vi "SVPO Vector Average Spectrum (Complex) (1 Ch).vi"(0 "complex spectrum [EU rms]":T7={"complex spectrum response"={"f0"=0.0, "df"=1.0, "complex spectrum"=[]}, "spectrum info"={"channel name"="", "description"="", "x-axis units"=0, "spectral info"={"spectrum type"=enum."Power [Magnitude^2]", "linear/dB"=enum."linear", "window"=0, "window size"=0, "FFT size"=0}, "engineering units"=0, "custom label"="", "dB reference [EU]"=0.0, "peak units"=enum."rms", "weighting filter"=0, "spectral density?"=FALSE, "unit label"="", "spectrum skewed?"=FALSE, "complimentary spectrum units"=enum."none"}} {"spectrum info"."x-axis units" items=["Time (s)"=0, "Frequency-CB (Hz)"=1, "Frequency-CPB (Hz)"=1248, "Frequency-Arbitrary (Hz)"=2357, "Quefrency (s)"=2, "Revolutions (rev)"=3, "Order"=4, "Speed (RPM)"=11, "Speed (rad/s)"=21, "Index"=65535]; "spectrum info"."weighting filter" items=["Linear", "A-weighting", "B-weighting", "C-weighting", "ITU-R 468-4", "Dolby", "CCITT", "C-message", "Wb", "Wc", "Wd", "We", "Wf", "Wh", "Wj", "Wk", "Wm", "AES17 20 kHz lowpass", "AES17 40 kHz lowpass", "AES17 20 kHz highpass", "AES17 40 kHz highpass"]; "spectrum info"."dB reference [EU]" format="%.2f"; "spectrum info"."engineering units" items=["custom..."=0, "V"=1, "A"=21, "C"=30, "pC"=31, "s"=32, "-"=29, "Pa"=2, "N"=20, "g"=3, "m/s^2"=4, "m/s"=5, "m"=6, "mm/s"=12, "mm"=13, "micron/s"=14, "micron"=15, "in/s^2"=7, "in/s"=8, "in"=9, "mil/s"=10, "mil"=11, "rad/s^2"=16, "rad/s"=17, "rad"=18, "deg/s^2"=26, "deg/s"=27, "deg"=28, "RPM"=22, "cycle/s^2"=23, "Hz"=24, "cycle"=25, "strain"=19]; "spectrum info"."spectral info"."window" items=["None "=0, "Hanning"=1, "Hamming"=2, "Blackman-Harris"=3, "Exact Blackman"=4, "Blackman"=5, "Flat Top"=6, "4 Term B-Harris "=7, "7 Term B-Harris"=8, "Low Sidelobe"=9, "Force - Exponential"=10, "Gaussian"=62]; "complex spectrum response"."complex spectrum" format="%.2f"; "complex spectrum response"."df" format="%.2f"; "complex spectrum response"."f0" format="%.2f"}, 3 "averaging weighting mode":enum16{"Linear", "Exponential"}(ring), 6 "exponential weight (10 %)":dbl=10.0 min=0.0 max=100.0 step=5.0, 9 "restart averaging (F)":bool) -> (13 "averages completed":dbl, 14 "average complex spectrum [EU rms]":T7={"complex spectrum response"={"f0"=0.0, "df"=1.0, "complex spectrum"=[]}, "spectrum info"={"channel name"="", "description"="", "x-axis units"=0, "spectral info"={"spectrum type"=enum."Power [Magnitude^2]", "linear/dB"=enum."linear", "window"=0, "window size"=0, "FFT size"=0}, "engineering units"=0, "custom label"="", "dB reference [EU]"=0.0, "peak units"=enum."rms", "weighting filter"=0, "spectral density?"=FALSE, "unit label"="", "spectrum skewed?"=FALSE, "complimentary spectrum units"=enum."none"}} {"spectrum info"."x-axis units" items=["Time (s)"=0, "Frequency-CB (Hz)"=1, "Frequency-CPB (Hz)"=1248, "Frequency-Arbitrary (Hz)"=2357, "Quefrency (s)"=2, "Revolutions (rev)"=3, "Order"=4, "Speed (RPM)"=11, "Speed (rad/s)"=21, "Index"=65535]; "spectrum info"."weighting filter" items=["Linear", "A-weighting", "B-weighting", "C-weighting", "ITU-R 468-4", "Dolby", "CCITT", "C-message", "Wb", "Wc", "Wd", "We", "Wf", "Wh", "Wj", "Wk", "Wm", "AES17 20 kHz lowpass", "AES17 40 kHz lowpass", "AES17 20 kHz highpass", "AES17 40 kHz highpass"]; "spectrum info"."dB reference [EU]" format="%.2f"; "spectrum info"."engineering units" items=["custom..."=0, "V"=1, "A"=21, "C"=30, "pC"=31, "s"=32, "-"=29, "Pa"=2, "N"=20, "g"=3, "m/s^2"=4, "m/s"=5, "m"=6, "mm/s"=12, "mm"=13, "micron/s"=14, "micron"=15, "in/s^2"=7, "in/s"=8, "in"=9, "mil/s"=10, "mil"=11, "rad/s^2"=16, "rad/s"=17, "rad"=18, "deg/s^2"=26, "deg/s"=27, "deg"=28, "RPM"=22, "cycle/s^2"=23, "Hz"=24, "cycle"=25, "strain"=19]; "spectrum info"."spectral info"."window" items=["None "=0, "Hanning"=1, "Hamming"=2, "Blackman-Harris"=3, "Exact Blackman"=4, "Blackman"=5, "Flat Top"=6, "4 Term B-Harris "=7, "7 Term B-Harris"=8, "Low Sidelobe"=9, "Force - Exponential"=10, "Gaussian"=62]; "complex spectrum response"."complex spectrum" format="%.2f"; "complex spectrum response"."df" format="%.2f"; "complex spectrum response"."f0" format="%.2f"})   [LabVIEW 2017]
doc: "Converts a frequency power spectrum to an order power spectrum. Use this VI to convert power spectrum results from constant-speed applications."
uses:
  <vilib>/addons/_NISVFA/_Shared subVIs/Controls/svc_Spectrum Info.ctl
  <vilib>/addons/_NISVFA/_Shared subVIs/Controls/svc_X-Axis Units.ctl
  <vilib>/addons/_NISVFA/_Shared subVIs/Controls/svc_Spectrum Type.ctl
  <vilib>/addons/_NISVFA/_Shared subVIs/Controls/svc_Engineering Units Text Ring.ctl
  <vilib>/addons/_NISVFA/_Shared subVIs/Controls/svc_Weighting Filter Text Ring.ctl
  <vilib>/addons/_NISVFA/_Shared subVIs/Controls/svc_Complimentary Spectrum Units.ctl
  <vilib>/addons/_NISVFA/_Shared subVIs/Spectrum Averaging/svpo_Average Array (complex).vi
  <vilib>/addons/_NISVFA/_Shared subVIs/Spectrum Info/svfa_Set Averaging Mode in Spectrum Info.vi
  <vilib>/addons/_NISVFA/_Shared subVIs/Spectrum Info/svfa_Get Averaging Mode from Spectrum Info.vi
  <vilib>/addons/_NISVFA/_Shared subVIs/Common/sv_Get NI Property Name String.vi
  <vilib>/addons/_NISVFA/_Shared subVIs/Spectrum Info/sfva_Set SV Info in Spectrum Info Description.vi
  <vilib>/addons/_NISVFA/_Shared subVIs/Spectrum Info/sfva_Get SV Info from Spectrum Info Description.vi
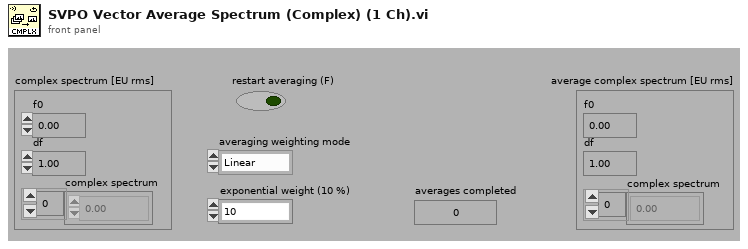
[diagram p1: front panel]
types:
  T1 = typedef "svc_Spectrum Info.ctl" = cluster{"channel name":string, "description":string, "x-axis units":T2, "spectral info":cluster{"spectrum type":T3, "linear/dB":enum16{"linear", "dB"}, "window":u16, "window size":i32, "FFT size":i32}, "engineering units":T4, "custom label":string, "dB reference [EU]":dbl, "peak units":enum16{"rms", "peak", "peak-peak"}, "weighting filter":T5, "spectral density?":bool, "unit label":string, "spectrum skewed?":bool, "complimentary spectrum units":T6}
  T2 = typedef "svc_X-Axis Units.ctl" = u16
  T3 = typedef "svc_Spectrum Type.ctl" = enum16{"FFT Spectrum [complex]", "Amplitude [Magnitude]", "Power [Magnitude^2]", "Cross Spectrum [complex]", "Frequency Response [Complex]"}
  T4 = typedef "svc_Engineering Units Text Ring.ctl" = u16
  T5 = typedef "svc_Weighting Filter Text Ring.ctl" = u16
  T6 = typedef "svc_Complimentary Spectrum Units.ctl" = enum16{"none", "radians", "degrees", "cycles", "imaginary"}
  T7 = cluster{"complex spectrum response":cluster{"f0":dbl, "df":dbl, "complex spectrum":cdb[]}, "spectrum info":T1}
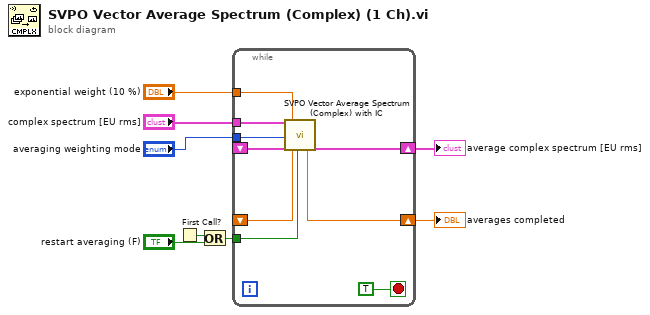
[diagram p0: block diagram]
diagram:
  n1 = First Call?() -> (First Call?: T/F=w3:bool)
  n2 = Or(x=w3, y="restart averaging (F)") -> (x .or. y?=w1:bool)
  n3 = while {
    tunnel: "complex spectrum [EU rms]" -> [w17]
    tunnel: "exponential weight (10 %)" -> [w16]
    tunnel: "averaging weighting mode" -> [w15]
    shift-right: [w14] -> w5
    shift-left: _ -> [w13]
    shift-right: [w11] -> w4
    shift-left: _ -> [w12]
    tunnel: w1 -> [w10]
    stop <- TRUE stop-if-true
    n4 = call <vilib>:"SVPO Vector Average Spectrum (Complex) with IC.vi"("complex spectrum [EU rms]"=w17, "averaging weighting mode"=w15, "average complex spectrum in"=w13, "exponential weight (10 %)"=w16, "averages completed in"=w12, "restart averaging (F)"=w10) -> ("averages completed out"=w11:dbl, "average complex spectrum out"=w14:T7)  [unwired: 12 in]
  }
  "average complex spectrum [EU rms]" <- w5
  "averages completed" <- w4
